vi "Get Step End Timestamp.vi"(8 "error in (no error)":errorcluster, 11 "Output Sequencer in":refnum<class "Output Sequencer.lvclass">) -> (0 "error out":errorcluster, 2 "Current Step End Timestamp":dbl, 3 "Output Sequencer out":refnum<class "Output Sequencer.lvclass">)   [LabVIEW 2020, in "Output Sequencer.lvlib" / "Output Sequencer.lvclass"]
uses:
  Output Sequencer.lvclass
  Output Sequencer.lvclass/Output Sequencer.ctl
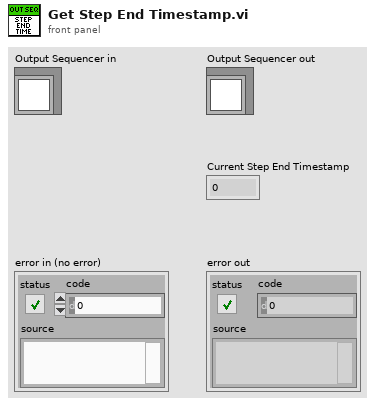
[diagram p1: front panel]
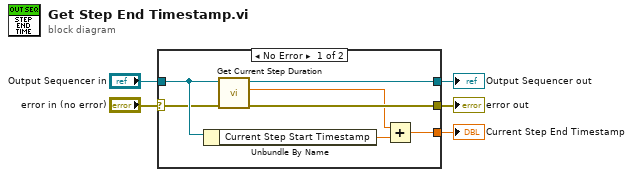
[diagram p0: block diagram]
diagram:
  n1 = case shown="No Error" "error in (no error)" {
    selector: "error in (no error)" -> [w6 w14]
    tunnel: [w12 w14] -> w5
    tunnel: [w11 w13] -> w4
    tunnel: [w10 _] -> w3
    tunnel: "Output Sequencer in" -> [w9 w13]
    frame No Error {
      n2 = Unbundle By Name(w9) -> ("Current Step Start Timestamp"=w7:dbl)
      n3 = call "Get Current Step Duration.vi"("error in (no error)"=w6, "Output Sequencer in"=w9) -> ("error out"=w12:errorcluster, "Duration"=w8:dbl, "Output Sequencer out"=w11:refnum<class "Output Sequencer.lvclass">)  [unwired: 7 in]
      n4 = Add(x=w8, y=w7) -> (x+y=w10:dbl)
    }
    frame Error {
    }
  }
  "error out" <- w5
  "Output Sequencer out" <- w4
  "Current Step End Timestamp" <- w3
